vi "Write Config.vi"(8 "error in (no error)":errorcluster caption="entrée d'erreur (pas d'erreur)", 10 "Config.lvclass":refnum<class "Config.lvclass">, 11 "GeneralFunctionality en entrée":refnum<class "GeneralFunctionality.lvclass">) -> (0 "error out":errorcluster caption="sortie d'erreur", 3 "GeneralFunctionality en sortie":refnum<class "GeneralFunctionality.lvclass">)   [LabVIEW 2020, in "GeneralFunctionality.lvclass"]
uses:
  GeneralFunctionality.lvclass
  Config/Config.lvclass
  GeneralFunctionality.lvclass/GeneralFunctionality.ctl
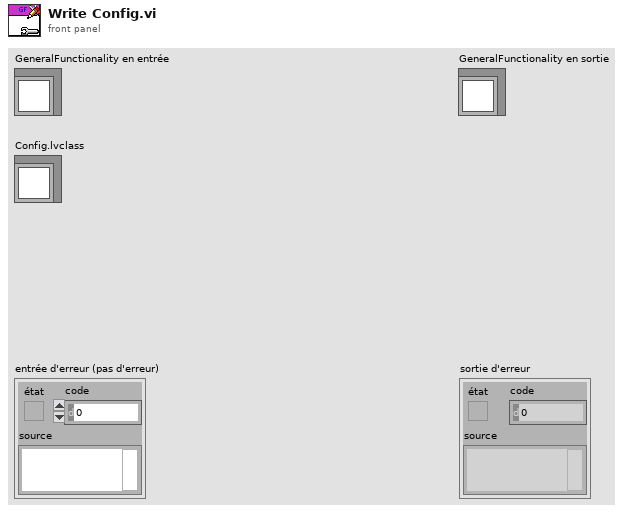
[diagram p1: front panel]
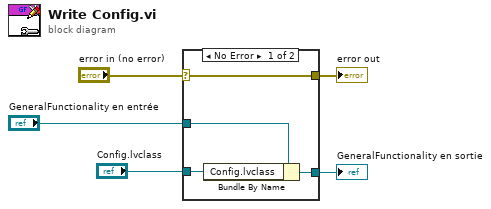
[diagram p0: block diagram]
diagram:
  n1 = case shown="No Error" "error in (no error)" {
    selector: "error in (no error)" -> [w9 w10]
    tunnel: [w9 w10] -> w4
    tunnel: [w7 w11] -> w2
    tunnel: "GeneralFunctionality en entrée" -> [w8 w11]
    tunnel: "Config.lvclass" -> [w6 _]
    frame No Error {
      n2 = Bundle By Name(cluster=w8, "Config.lvclass"=w6) -> (w7:refnum<class "GeneralFunctionality.lvclass">)
    }
    frame Error {
    }
  }
  "error out" <- w4
  "GeneralFunctionality en sortie" <- w2
